vi "Main.vi"(8 "error in (no error)":errorcluster, 11 "DAQMH121119OrcaFlashBase in":refnum<class "DAQOrcaFlash.lvclass">) -> (0 "error out":errorcluster, 3 "component":refnum<class "DAQOrcaFlash.lvclass">)   [LabVIEW 2012, in "DAQOrcaFlash.lvclass"]
doc: "Main VI of the component."
uses:
  DAQOrcaFlash.lvclass
  binning.ctl
  DAQOrcaFlash.lvclass/DAQOrcaFlash.ctl
  <vilib>/Distrio/Murmex/InitialiseMessage/InitialiseMessage.lvclass
  <vilib>/Distrio/Murmex/Murmex/command_enum.ctl
  <vilib>/Distrio/Murmex/TerminateMessage/TerminateMessage.lvclass
  <vilib>/Distrio/Murmex/StartMessage/run mode enum.ctl
  <vilib>/Distrio/Murmex/StopMessage/StopMessage.lvclass
  <vilib>/Distrio/Murmex/StartMessage/StartMessage.lvclass
  <vilib>/Distrio/Murmex/ConfigureMessage/ConfigureMessage.lvclass
  <vilib>/Distrio/Murmex/Murmex/update_cluster.ctl
  class variable.vi
  <vilib>/Distrio/Murmex/Murmex/Set VI reference.vi
  <vilib>/Distrio/Murmex/Murmex/Set log reference.vi
  <vilib>/Distrio/Murmex/Murmex/Set configure at initialise.vi
  <vilib>/Distrio/Murmex/Murmex/Set relay start stop to observers.vi
  <vilib>/Distrio/Murmex/Murmex/Murmex.lvclass
  <vilib>/Distrio/Murmex/Message/Message.lvclass
panel:
  in  "button:configure":bool
  in  "button:quit":bool
  in  "terminate?":bool
  out "progress bar":sgl(slide) scale=0.0..1.0
  in  "Tab":T1(tab)
  in  "Rolling shutter pace":sgl[unit]=9.74436e-06 min=9.74436e-06 max=10 step=3.76e-09 format="%#_7g"
  out "Frames per second":dbl[unit]
  out "Virtual slit width":dbl[unit]
  in  "button:start_sweep":bool
  in  "y offset":u16 max=2048 step=4
  in  "x offset":u16 max=2048 step=4
  in  "y resolution":u16=2048 min=4 max=2048 step=4
  in  "x resolution":u16=2048 min=4 max=2048 step=4
  in  "binning":T2=1 items=["1x1"=1, "2x2"=2, "4x4"=4]
  in  "no. of frames":i32=1 min=1 step=1
  in  "line exposure time":dbl[unit]=0.1 caption="exposure time"
  in  "button:start focus":bool
  in  "File name":string
  in  "Subfolder levels":string[](array[string])
  in  "Custom saving path":bool
  in  "directory out":path
  in  "button:convert":bool
  out "filename":string
  in  "directory in":path
  in  "ID":string="orca"
  in  "log":string
  in  "button:AO":bool
  # "Convert here properietary file formats of Hamamatsu to TIFF format."
  # "Calculates the merit factor, \nused for Adaptive Optics (AO)"
  # "DAQMH121119OrcaFlash\n\nImplemented by:\nMarcel van 't Hoff\nUniversity of Florence, Ital\n\nThis component support only the Hamamatsu Orca Flash 4.0"
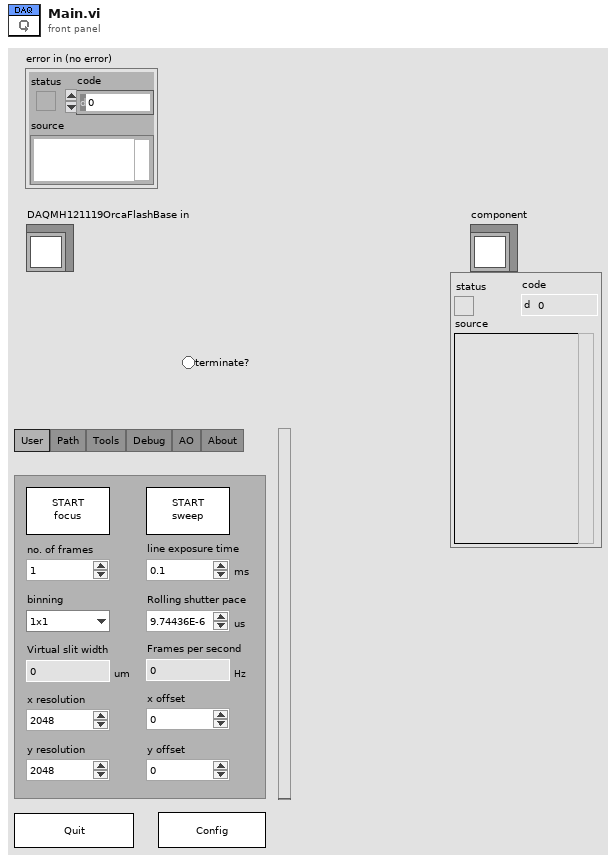
[diagram p1: front panel]
types:
  T1 = enum32{"User", "Path", "Tools", "Debug", "AO", "About"}
  T2 = typedef "DAQOrcaFlash.lvclass/binning.ctl" = u16
  T3 = typedef "Murmex.lvlib/Murmex.lvclass/command_enum.ctl" = enum16{"null", "initialise", "reset", "terminate", "acknowledge", "update", "inspect", "inform", "proceed", "start", "stop", "fetch", "configure", "generic"}
  T4 = typedef "Murmex.lvlib/StartMessage.lvclass/run mode enum.ctl" = enum16{"infinite", "finite"}
  T5 = typedef "Murmex.lvlib/Murmex.lvclass/update_cluster.ctl" = cluster{"target ID":string, "key chains":string[], "values":variant[]}
  T6 = enum8{"Enabled", "Disabled", "Disabled and Grayed Out"}
  T7 = typedef "Murmex.lvclass/command_enum.ctl" = enum16{"null", "initialise", "reset", "terminate", "acknowledge", "update", "inspect", "inform", "proceed", "start", "stop", "fetch", "configure", "generic"}
  T8 = typedef "Murmex.lvclass/Event type enumerations.ctl" = enum16{"before", "after"}
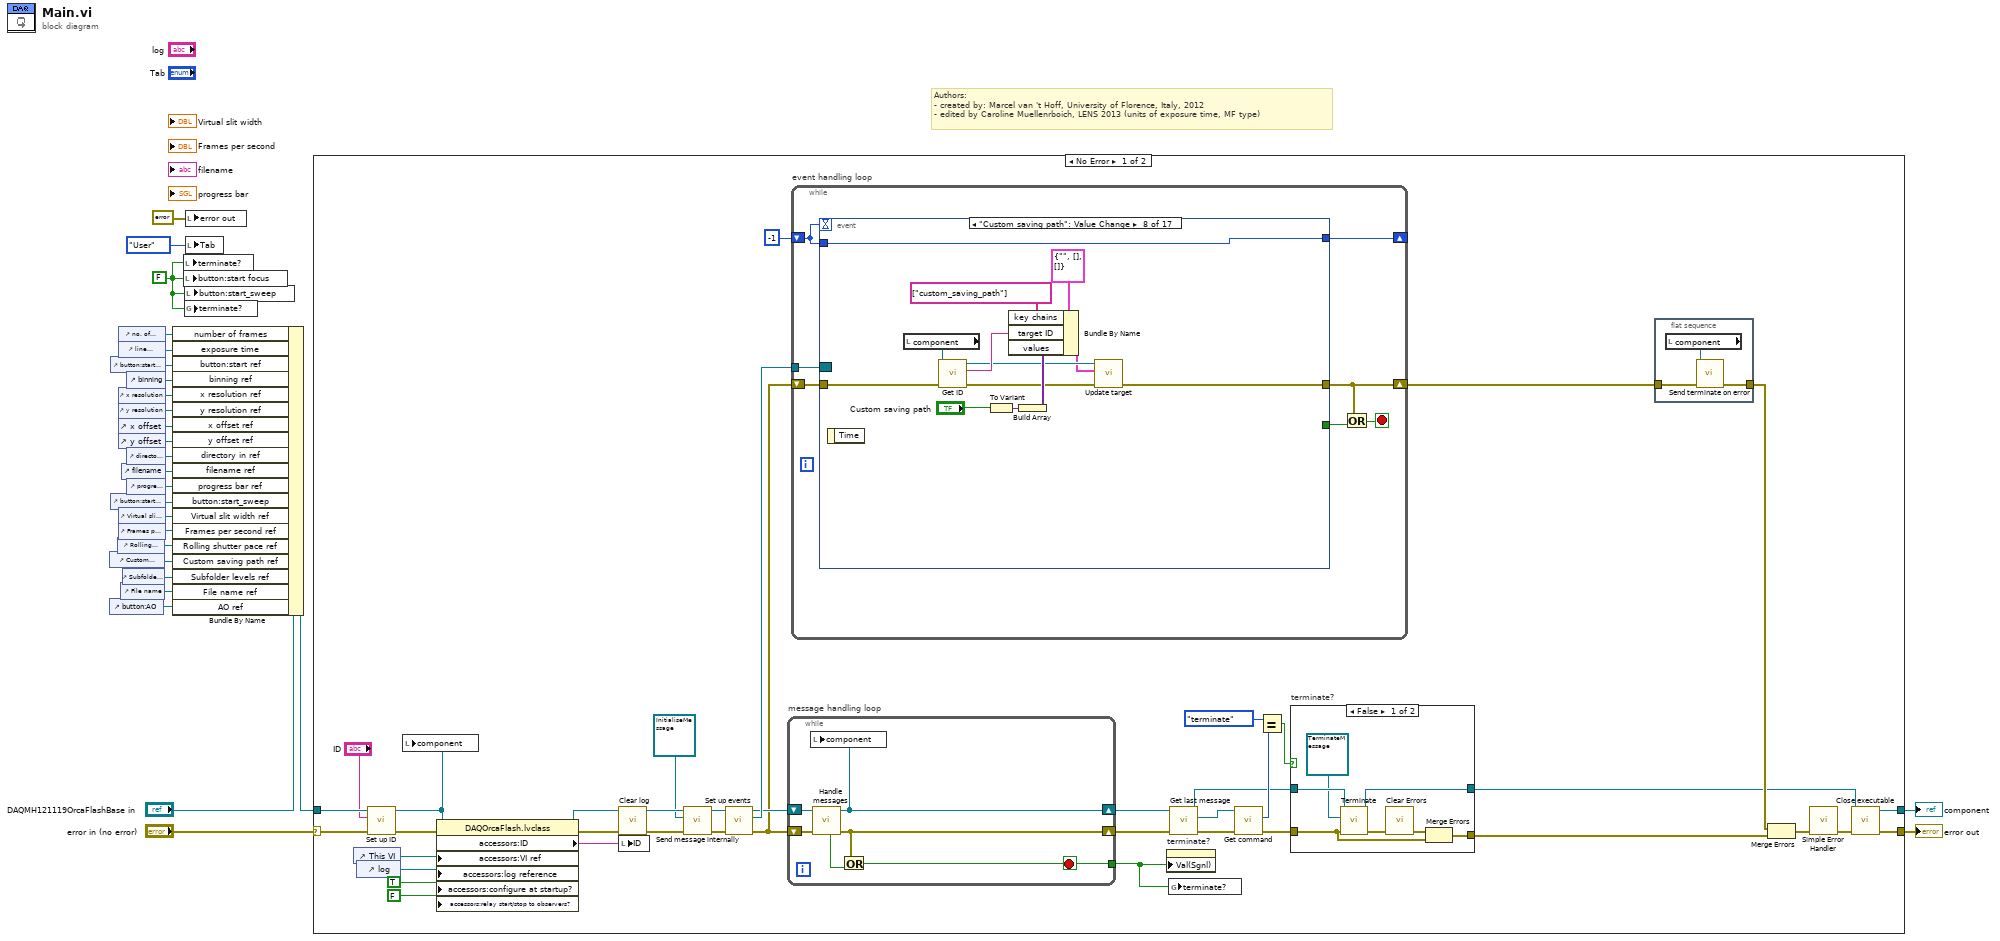
[diagram p0: block diagram]
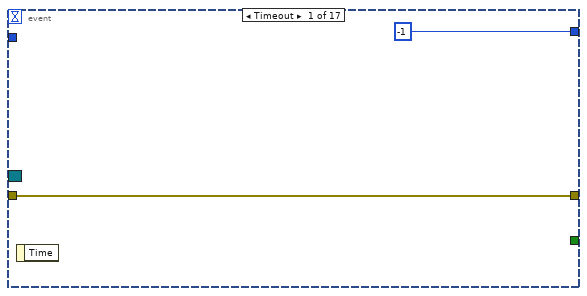
[diagram p3: hidden frame]
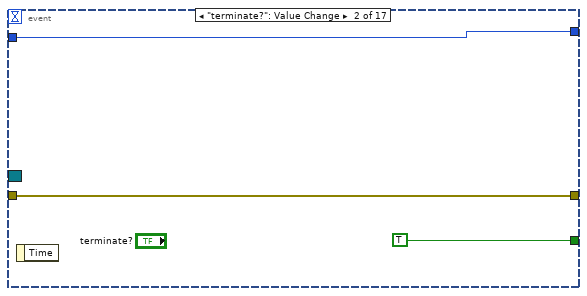
[diagram p4: hidden frame]
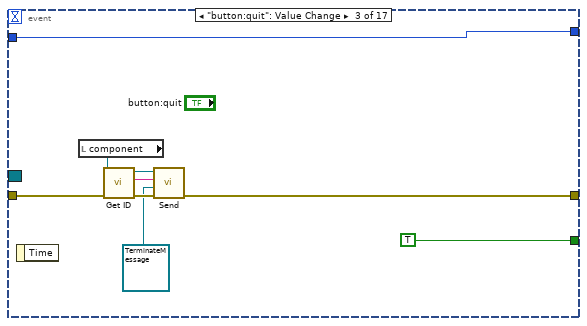
[diagram p5: hidden frame]
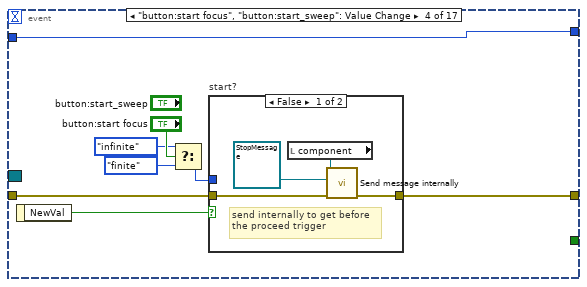
[diagram p6: hidden frame]
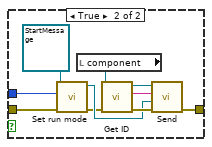
[diagram p7: hidden frame]
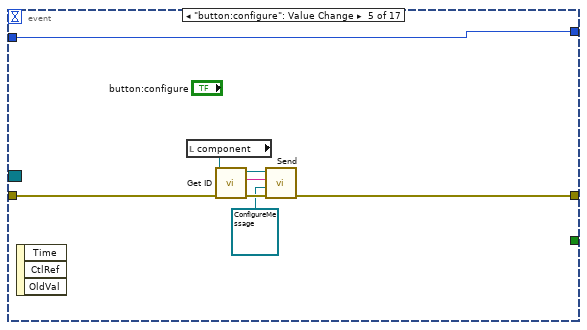
[diagram p8: hidden frame]
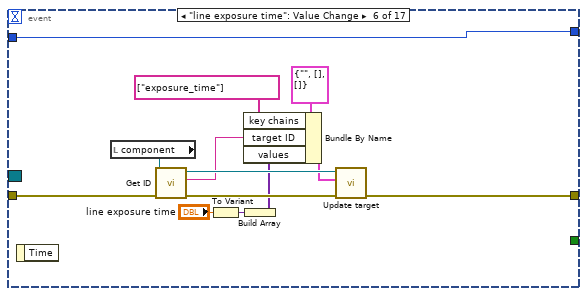
[diagram p9: hidden frame]
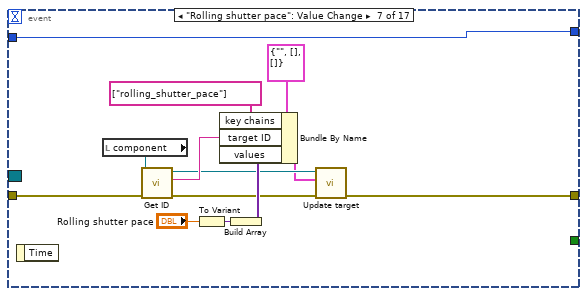
[diagram p10: hidden frame]
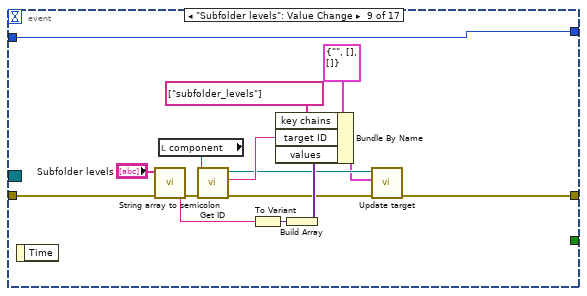
[diagram p11: hidden frame]
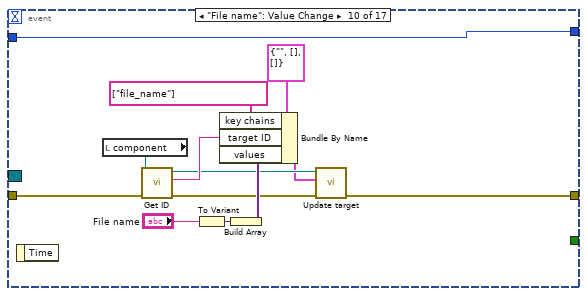
[diagram p12: hidden frame]
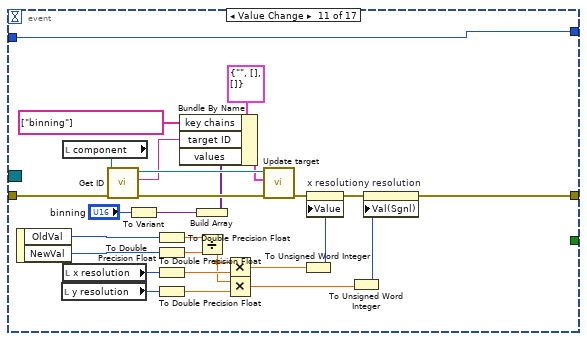
[diagram p13: hidden frame]
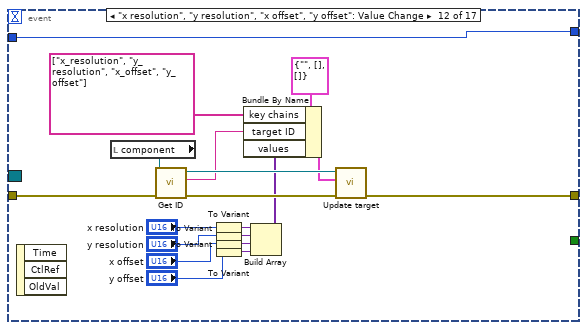
[diagram p14: hidden frame]
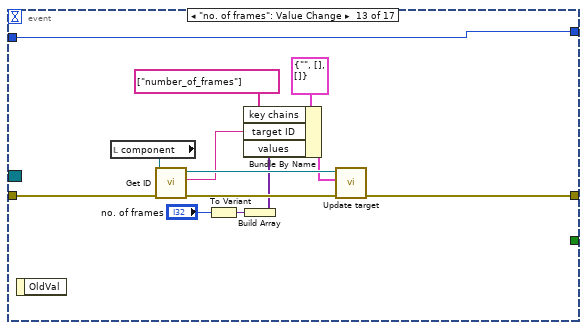
[diagram p15: hidden frame]
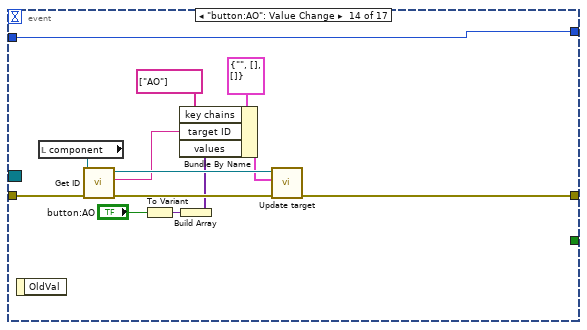
[diagram p16: hidden frame]
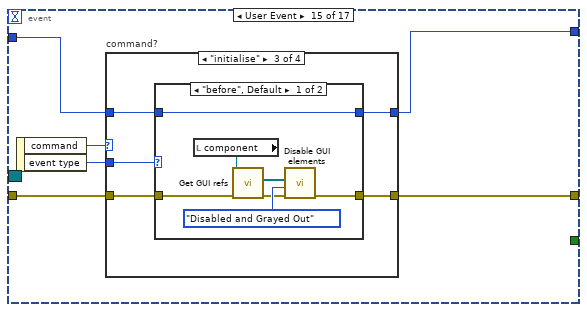
[diagram p17: hidden frame]
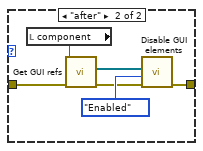
[diagram p19: hidden frame]
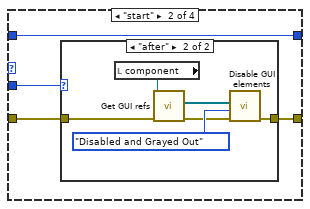
[diagram p20: hidden frame]
diagram:
  w9 = FALSE ("terminate?")
  # "Authors: \n- created by: Marcel van 't Hoff, University of Florence, Italy, 2012\n- edited by Caroline Muellenrboich, LENS 2013 (units of exposure time, MF type)"
  n1 = control-ref of="button:AO"() -> (w1:refnum<vi>)
  n2 = control-ref of="Custom saving path"() -> (w3:refnum<vi>)
  n3 = control-ref of="button:start focus"() -> (w20:refnum<vi>)
  n4 = control-ref of="button:start_sweep"() -> (w10:refnum<vi>)
  n5 = control-ref of="Rolling shutter pace"() -> (w6:refnum<vi>)
  n6 = control-ref of="no. of frames"() -> (w21:refnum<vi>)
  n7 = control-ref of="line exposure time"() -> (w22:refnum<vi>)
  n8 = control-ref of="x resolution"() -> (w18:refnum<vi>)
  n9 = control-ref of="y resolution"() -> (w17:refnum<vi>)
  n10 = control-ref of="x offset"() -> (w16:refnum<vi>)
  n11 = control-ref of="y offset"() -> (w15:refnum<vi>)
  n12 = control-ref of="Virtual slit width"() -> (w8:refnum<vi>)
  n13 = control-ref of="Frames per second"() -> (w7:refnum<vi>)
  n14 = control-ref of="File name"() -> (w5:refnum<vi>)
  n15 = control-ref of="filename"() -> (w13:refnum<vi>)
  n16 = control-ref of="Subfolder levels"() -> (w4:refnum<vi>)
  n17 = control-ref of="binning"() -> (w19:refnum<vi>)
  n18 = control-ref of="directory in"() -> (w14:refnum<vi>)
  n19 = control-ref of="progress bar"() -> (w12:refnum<vi>)
  n20 = Bundle By Name(cluster="DAQMH121119OrcaFlashBase in", "number of frames"=w21, "exposure time"=w22, "button:start ref"=w20, "binning ref"=w19, "x resolution ref"=w18, "y resolution ref"=w17, "x offset ref"=w16, "y offset ref"=w15, "directory in ref"=w14, "filename ref"=w13, "progress bar ref"=w12, "button:start_sweep"=w10, "Virtual slit width ref"=w8, "Frames per second ref"=w7, "Rolling shutter pace ref"=w6, "Custom saving path ref"=w3, "Subfolder levels ref"=w4, "File name ref"=w5, "AO ref"=w1) -> (w23:refnum<class "DAQOrcaFlash.lvclass">)
  n21 = local write "terminate?"(w9) -> ()
  n22 = local write "button:start focus"(w9) -> ()
  n23 = local write "button:start_sweep"(w9) -> ()
  n24 = global write "class variable.vi" "terminate?"(w9) -> ()
  n25 = local write "error out"(errorcluster {"status"=FALSE, "code"=0, "source"=""} ("error out")) -> ()
  n26 = local write "Tab"(T1."User" ("Tab")) -> ()
  n27 = case shown="No Error" "error in (no error)" {
    selector: "error in (no error)" -> [w60 w340]
    tunnel: [w55 w340] -> w26
    tunnel: [w54 w339] -> w25
    tunnel: w23 -> [w61 w339]
    frame No Error {
      n28 = control-ref of="This VI"() -> (w50:refnum<vi>)
      n29 = control-ref of="log"() -> (w49:refnum<vi>)
      n30 = call <vilib>:"Set up ID.vi"("error in (no error)"=w60, "component ID"="ID", "MurmexBase in"=w61) -> ("error out"=w52:errorcluster, "MurmexBase out"=w40:refnum<class "DAQOrcaFlash.lvclass">)  [unwired: 6 in, 1 out]
      n31 = local write "component"(w40) -> ()
      n32 = property class="DAQOrcaFlash.lvclass"(reference=w40, error in=w52, "accessors:VI ref"=w50, "accessors:log reference"=w49, "accessors:configure at startup?"=TRUE ("configure at startup?"), "accessors:relay start/stop to observers?"=FALSE ("relay start/stop to observers?")) -> (reference out=w47:refnum<class "DAQOrcaFlash.lvclass">, error out=w48:errorcluster, "accessors:ID"=w51:string)
      n33 = call <vilib>:"Clear log.vi"("error in (no error)"=w48, "MurmexBase in"=w47) -> ("error out"=w62:errorcluster, "MurmexBase out"=w66:refnum<class "DAQOrcaFlash.lvclass">)  [unwired: 8 in]
      n34 = local write "ID"(w51) -> ()
      n35 = call <vilib>:"Send message internally.vi"("error in (no error)"=w62, "Message"=refnum<class "InitialiseMessage.lvclass"> refnum ("Distrio Murmex 1.0:InitialiseMessage"), "Murmex in"=w66) -> ("error out"=w58:errorcluster, "Murmex out"=w57:refnum<class "DAQOrcaFlash.lvclass">)  [unwired: 7 in]
      n36 = call <vilib>:"Set up events.vi"("error in (no error)"=w58, "MurmexBase in"=w57) -> ("error out"=w29:errorcluster, "Event Registration Refnum"=w64:refnum<event-registration>, "MurmexBase out"=w31:refnum<class "DAQOrcaFlash.lvclass">)  [unwired: 7 in]
      n37 = while "message handling loop" {
        shift-right: [w334] -> w37
        shift-left: w29 -> [w336]
        shift-right: [w333] -> w39
        shift-left: w31 -> [w338]
        tunnel: [w335] -> w30
        stop <- w335 stop-if-true
        n38 = call <vilib>:"Handle messages.vi"("error in (no error)"=w336, "Murmex in"=w338) -> ("error out"=w334:errorcluster, "Murmex out"=w333:refnum<class "DAQOrcaFlash.lvclass">, "terminated?"=w337:bool)  [unwired: 7 in]
        n39 = local write "component"(w333) -> ()
        n40 = Or(x=w334, y=w337) -> (x .or. y?=w335:bool)
      }
      n41 = while "event handling loop" {
        shift-right: [w85] -> _
        shift-left: -1 -> [w84]
        tunnel: w64 -> [w82]
        shift-right: [w81] -> w63
        shift-left: w29 -> [w83]
        stop <- w79 stop-if-true
        n42 = event shown="[7] \"Custom saving path\": Value Change" {
          selector: w82 -> [_ _ _ _ _ _ _ _ _ _ _ _ _ _ _ _ _]
          dyn-events: _ -> [_ _ _ _ _ _ _ _ _ _ _ _ _ _ _ _ _]
          timeout: w84 -> [_ _ _ _ _ _ _ _ _ _ _ _ _ _ _ _ _]
          tunnel: [-1 w90 w99 w107 w129 w142 w155 w168 w183 w196 w224 w243 w256 w269 w271 w321 w332] -> w85
          tunnel: w84 -> [_ w90 w99 w107 w129 w142 w155 w168 w183 w196 w224 w243 w256 w269 w272 w321 w332]
          tunnel: w83 -> [w86 w89 w92 w106 w125 w141 w154 w167 w172 w195 w223 w242 w255 w268 w273 w320 w329]
          tunnel: [w86 w89 w94 w105 w124 w140 w147 w156 w176 w188 w206 w241 w254 w257 w274 w319 w322] -> w81
          tunnel: [_ TRUE TRUE _ _ _ _ _ _ _ _ _ _ _ _ _ _] -> w80
          event Timeout {
            n43 = event-data() -> ()  [unwired: 1 in, 1 out]
          }
          event "terminate?": Value Change {
            n44 = event-data() -> ()  [unwired: 1 in, 1 out]
          }
          event "button:quit": Value Change {
            n45 = event-data() -> ()  [unwired: 1 in, 1 out]
            n46 = local read "component"() -> (w97:refnum<class "DAQOrcaFlash.lvclass">)
            n47 = call <vilib>:"Get ID.vi"("error in (no error)"=w92, "Murmex in"=w97) -> ("error out"=w93:errorcluster, "component id"=w95:string, "Murmex out"=w96:refnum<class "DAQOrcaFlash.lvclass">)  [unwired: 7 in]
            n48 = call <vilib>:"Send.vi"("error in (no error)"=w93, "Message"=refnum<class "TerminateMessage.lvclass"> refnum ("Message in"), "recipient"=w95, "Murmex in"=w96) -> ("error out"=w94:errorcluster)  [unwired: 6 in, 1 out]
          }
          event "button:start focus", "button:start_sweep": Value Change {
            n49 = event-data() -> ("NewVal"=w102:bool)  [unwired: 1 in]
            n50 = Select(t=run_mode_enum."infinite" ("run mode"), s="button:start focus", f=run_mode_enum."finite" ("run mode")) -> (s? t:f=w103:T4)
            n51 = case "start?" shown="False" w102 {
              tunnel: [w110 w117] -> w105
              tunnel: w106 -> [w111 w114]
              tunnel: w103 -> [_ w112]
              frame False {
                # "send internally to get before\nthe proceed trigger"
                n52 = local read "component"() -> (w109:refnum<class "DAQOrcaFlash.lvclass">)
                n53 = call <vilib>:"Send message internally.vi"("error in (no error)"=w111, "Message"=refnum<class "StopMessage.lvclass"> refnum ("Distrio Murmex 1.0:StopMessage"), "Murmex in"=w109) -> ("error out"=w110:errorcluster)  [unwired: 7 in, 1 out]
              }
              frame True {
                n54 = call <vilib>:"Set run mode.vi"("error in (no error)"=w114, "run mode"=w112, "StartMessage in"=refnum<class "StartMessage.lvclass"> refnum ("Distrio Murmex 1.0:StartMessage")) -> ("error out"=w113:errorcluster, "StartMessage out"=w115:refnum<class "StartMessage.lvclass">)  [unwired: 7 in]
                n55 = local read "component"() -> (w121:refnum<class "DAQOrcaFlash.lvclass">)
                n56 = call <vilib>:"Get ID.vi"("error in (no error)"=w113, "Murmex in"=w121) -> ("error out"=w118:errorcluster, "component id"=w119:string, "Murmex out"=w120:refnum<class "DAQOrcaFlash.lvclass">)  [unwired: 7 in]
                n57 = call <vilib>:"Send.vi"("error in (no error)"=w118, "Message"=w115, "recipient"=w119, "Murmex in"=w120) -> ("error out"=w117:errorcluster)  [unwired: 6 in, 1 out]
              }
            }
          }
          event "button:configure": Value Change {
            n58 = event-data() -> ()  [unwired: 1 in, 3 out]
            n59 = local read "component"() -> (w123:refnum<class "DAQOrcaFlash.lvclass">)
            n60 = call <vilib>:"Get ID.vi"("error in (no error)"=w125, "Murmex in"=w123) -> ("error out"=w126:errorcluster, "component id"=w127:string, "Murmex out"=w128:refnum<class "DAQOrcaFlash.lvclass">)  [unwired: 7 in]
            n61 = call <vilib>:"Send.vi"("error in (no error)"=w126, "Message"=refnum<class "ConfigureMessage.lvclass"> refnum ("ConfigureMessage"), "recipient"=w127, "Murmex in"=w128) -> ("error out"=w124:errorcluster)  [unwired: 6 in, 1 out]
          }
          event "line exposure time": Value Change {
            n62 = event-data() -> ()  [unwired: 1 in, 1 out]
            n63 = local read "component"() -> (w139:refnum<class "DAQOrcaFlash.lvclass">)
            n64 = call <vilib>:"Get ID.vi"("error in (no error)"=w141, "Murmex in"=w139) -> ("error out"=w137:errorcluster, "component id"=w134:string, "Murmex out"=w138:refnum<class "DAQOrcaFlash.lvclass">)  [unwired: 7 in]
            n65 = To Variant(anything="line exposure time") -> (Variant=w132:variant)
            n66 = Build Array(w132) -> (w131:variant[])
            n67 = Bundle By Name(cluster=T5 {"target ID"="", "key chains"=[], "values"=[]} ("update cluster"), "key chains"=string[] ["exposure_time"], "target ID"=w134, "values"=w131) -> (w135:T5)
            n68 = call <vilib>:"Update target.vi"("error in (no error)"=w137, "update cluster"=w135, "MurmexBase in"=w138) -> ("error out"=w140:errorcluster)  [unwired: 7 in, 1 out]
          }
          event "Rolling shutter pace": Value Change {
            n69 = event-data() -> ()  [unwired: 1 in, 1 out]
            n70 = local read "component"() -> (w152:refnum<class "DAQOrcaFlash.lvclass">)
            n71 = call <vilib>:"Get ID.vi"("error in (no error)"=w154, "Murmex in"=w152) -> ("error out"=w148:errorcluster, "component id"=w151:string, "Murmex out"=w146:refnum<class "DAQOrcaFlash.lvclass">)  [unwired: 7 in]
            n72 = To Variant(anything="Rolling shutter pace") -> (Variant=w153:variant)
            n73 = Build Array(w153) -> (w149:variant[])
            n74 = Bundle By Name(cluster=T5 {"target ID"="", "key chains"=[], "values"=[]} ("update cluster"), "key chains"=string[] ["rolling_shutter_pace"], "target ID"=w151, "values"=w149) -> (w144:T5)
            n75 = call <vilib>:"Update target.vi"("error in (no error)"=w148, "update cluster"=w144, "MurmexBase in"=w146) -> ("error out"=w147:errorcluster)  [unwired: 7 in, 1 out]
          }
          event "Custom saving path": Value Change {
            n76 = event-data() -> ()  [unwired: 1 in, 1 out]
            n77 = local read "component"() -> (w165:refnum<class "DAQOrcaFlash.lvclass">)
            n78 = call <vilib>:"Get ID.vi"("error in (no error)"=w167, "Murmex in"=w165) -> ("error out"=w161:errorcluster, "component id"=w164:string, "Murmex out"=w160:refnum<class "DAQOrcaFlash.lvclass">)  [unwired: 7 in]
            n79 = To Variant(anything="Custom saving path") -> (Variant=w166:variant)
            n80 = Build Array(w166) -> (w162:variant[])
            n81 = Bundle By Name(cluster=T5 {"target ID"="", "key chains"=[], "values"=[]} ("update cluster"), "key chains"=string[] ["custom_saving_path"], "target ID"=w164, "values"=w162) -> (w158:T5)
            n82 = call <vilib>:"Update target.vi"("error in (no error)"=w161, "update cluster"=w158, "MurmexBase in"=w160) -> ("error out"=w156:errorcluster)  [unwired: 7 in, 1 out]
          }
          event "Subfolder levels": Value Change {
            n83 = event-data() -> ()  [unwired: 1 in, 1 out]
            n84 = call "String array to semicolon.vi"("error in"=w172, "String array"="Subfolder levels") -> ("error out"=w171:errorcluster, "Semicolon string"=w170:string)  [unwired: 8 in]
            n85 = local read "component"() -> (w181:refnum<class "DAQOrcaFlash.lvclass">)
            n86 = call <vilib>:"Get ID.vi"("error in (no error)"=w171, "Murmex in"=w181) -> ("error out"=w177:errorcluster, "component id"=w180:string, "Murmex out"=w175:refnum<class "DAQOrcaFlash.lvclass">)  [unwired: 7 in]
            n87 = To Variant(anything=w170) -> (Variant=w182:variant)
            n88 = Build Array(w182) -> (w178:variant[])
            n89 = Bundle By Name(cluster=T5 {"target ID"="", "key chains"=[], "values"=[]} ("update cluster"), "key chains"=string[] ["subfolder_levels"], "target ID"=w180, "values"=w178) -> (w173:T5)
            n90 = call <vilib>:"Update target.vi"("error in (no error)"=w177, "update cluster"=w173, "MurmexBase in"=w175) -> ("error out"=w176:errorcluster)  [unwired: 7 in, 1 out]
          }
          event "File name": Value Change {
            n91 = event-data() -> ()  [unwired: 1 in, 1 out]
            n92 = local read "component"() -> (w193:refnum<class "DAQOrcaFlash.lvclass">)
            n93 = call <vilib>:"Get ID.vi"("error in (no error)"=w195, "Murmex in"=w193) -> ("error out"=w189:errorcluster, "component id"=w192:string, "Murmex out"=w187:refnum<class "DAQOrcaFlash.lvclass">)  [unwired: 7 in]
            n94 = To Variant(anything="File name") -> (Variant=w194:variant)
            n95 = Build Array(w194) -> (w190:variant[])
            n96 = Bundle By Name(cluster=T5 {"target ID"="", "key chains"=[], "values"=[]} ("update cluster"), "key chains"=string[] ["file_name"], "target ID"=w192, "values"=w190) -> (w185:T5)
            n97 = call <vilib>:"Update target.vi"("error in (no error)"=w189, "update cluster"=w185, "MurmexBase in"=w187) -> ("error out"=w188:errorcluster)  [unwired: 7 in, 1 out]
          }
          event Value Change {
            n98 = event-data() -> ("OldVal"=w201:T2, "NewVal"=w200:T2)  [unwired: 1 in]
            n99 = local read "y resolution"() -> (w214:u16)
            n100 = local read "component"() -> (w222:refnum<class "DAQOrcaFlash.lvclass">)
            n101 = local read "x resolution"() -> (w213:u16)
            n102 = call <vilib>:"Get ID.vi"("error in (no error)"=w223, "Murmex in"=w222) -> ("error out"=w220:errorcluster, "component id"=w217:string, "Murmex out"=w221:refnum<class "DAQOrcaFlash.lvclass">)  [unwired: 7 in]
            n103 = To Variant(anything="binning") -> (Variant=w209:variant)
            n104 = To Double Precision Float(number=w201) -> (double precision float=w199:dbl)
            n105 = To Double Precision Float(number=w200) -> (double precision float=w198:dbl)
            n106 = To Double Precision Float(number=w213) -> (double precision float=w210:dbl)
            n107 = To Double Precision Float(number=w214) -> (double precision float=w211:dbl)
            n108 = Build Array(w209) -> (w215:variant[])
            n109 = Bundle By Name(cluster=T5 {"target ID"="", "key chains"=[], "values"=[]} ("update cluster"), "key chains"=string[] ["binning"], "target ID"=w217, "values"=w215) -> (w218:T5)
            n110 = Divide(x=w199, y=w198) -> (x/y=w197:dbl)
            n111 = Multiply(x=w197, y=w210) -> (x*y=w207:dbl)
            n112 = Multiply(x=w197, y=w211) -> (x*y=w208:dbl)
            n113 = call <vilib>:"Update target.vi"("error in (no error)"=w220, "update cluster"=w218, "MurmexBase in"=w221) -> ("error out"=w205:errorcluster)  [unwired: 7 in, 1 out]
            n114 = To Unsigned Word Integer(number=w207) -> (unsigned 16bit integer=w204:u16)
            n115 = property on="x resolution" class="DigNum (strict)"(error in=w205, "Value"=w204) -> (error out=w202:errorcluster)  [unwired: 1 in, 1 out]
            n116 = To Unsigned Word Integer(number=w208) -> (unsigned 16bit integer=w203:u16)
            n117 = property on="y resolution" class="DigNum (strict)"(error in=w202, "Val(Sgnl)"=w203) -> (error out=w206:errorcluster)  [unwired: 1 in, 1 out]
          }
          event "x resolution", "y resolution", "x offset", "y offset": Value Change {
            n118 = event-data() -> ()  [unwired: 1 in, 3 out]
            n119 = local read "component"() -> (w240:refnum<class "DAQOrcaFlash.lvclass">)
            n120 = call <vilib>:"Get ID.vi"("error in (no error)"=w242, "Murmex in"=w240) -> ("error out"=w238:errorcluster, "component id"=w235:string, "Murmex out"=w239:refnum<class "DAQOrcaFlash.lvclass">)  [unwired: 7 in]
            n121 = To Variant(anything="x resolution") -> (Variant=w228:variant)
            n122 = To Variant(anything="y resolution") -> (Variant=w227:variant)
            n123 = To Variant(anything="x offset") -> (Variant=w226:variant)
            n124 = To Variant(anything="y offset") -> (Variant=w225:variant)
            n125 = Build Array(w228, w227, w226, w225) -> (w229:variant[])
            n126 = Bundle By Name(cluster=T5 {"target ID"="", "key chains"=[], "values"=[]} ("update cluster"), "key chains"=string[] ["x_resolution", "y_resolution", "x_offset", "y_offset"], "target ID"=w235, "values"=w229) -> (w236:T5)
            n127 = call <vilib>:"Update target.vi"("error in (no error)"=w238, "update cluster"=w236, "MurmexBase in"=w239) -> ("error out"=w241:errorcluster)  [unwired: 7 in, 1 out]
          }
          event "no. of frames": Value Change {
            n128 = event-data() -> ()  [unwired: 1 in, 1 out]
            n129 = local read "component"() -> (w253:refnum<class "DAQOrcaFlash.lvclass">)
            n130 = call <vilib>:"Get ID.vi"("error in (no error)"=w255, "Murmex in"=w253) -> ("error out"=w251:errorcluster, "component id"=w248:string, "Murmex out"=w252:refnum<class "DAQOrcaFlash.lvclass">)  [unwired: 7 in]
            n131 = To Variant(anything="no. of frames") -> (Variant=w244:variant)
            n132 = Build Array(w244) -> (w246:variant[])
            n133 = Bundle By Name(cluster=T5 {"target ID"="", "key chains"=[], "values"=[]} ("update cluster"), "key chains"=string[] ["number_of_frames"], "target ID"=w248, "values"=w246) -> (w249:T5)
            n134 = call <vilib>:"Update target.vi"("error in (no error)"=w251, "update cluster"=w249, "MurmexBase in"=w252) -> ("error out"=w254:errorcluster)  [unwired: 7 in, 1 out]
          }
          event "button:AO": Value Change {
            n135 = event-data() -> ()  [unwired: 1 in, 1 out]
            n136 = local read "component"() -> (w267:refnum<class "DAQOrcaFlash.lvclass">)
            n137 = call <vilib>:"Get ID.vi"("error in (no error)"=w268, "Murmex in"=w267) -> ("error out"=w265:errorcluster, "component id"=w258:string, "Murmex out"=w266:refnum<class "DAQOrcaFlash.lvclass">)  [unwired: 7 in]
            n138 = To Variant(anything="button:AO") -> (Variant=w260:variant)
            n139 = Build Array(w260) -> (w261:variant[])
            n140 = Bundle By Name(cluster=T5 {"target ID"="", "key chains"=[], "values"=[]} ("update cluster"), "key chains"=string[] ["AO"], "target ID"=w258, "values"=w261) -> (w263:T5)
            n141 = call <vilib>:"Update target.vi"("error in (no error)"=w265, "update cluster"=w263, "MurmexBase in"=w266) -> ("error out"=w257:errorcluster)  [unwired: 7 in, 1 out]
          }
          event User Event {
            n142 = event-data() -> ("command"=w275:T7, "event type"=w270:T8)  [unwired: 1 in]
            n143 = case "command?" shown="\"initialise\"" w275 {
              tunnel: [w279 w290 w301 w315] -> w274
              tunnel: w273 -> [w278 w289 w302 w315]
              tunnel: [w277 w288 w300 w314] -> w271
              tunnel: w272 -> [w277 w288 w299 w314]
              tunnel: w270 -> [w276 w287 w298 _]
              frame "stop" {
                n144 = case shown="\"before\", Default" w276 {
                  tunnel: [w280 w286] -> w279
                  tunnel: w278 -> [w280 w283]
                  frame "before", Default {
                  }
                  frame "after" {
                    n145 = local read "component"() -> (w284:refnum<class "DAQOrcaFlash.lvclass">)
                    n146 = call "Get GUI refs.vi"("error in (no error)"=w283, "DAQMH121119OrcaFlash in"=w284) -> ("error out"=w282:errorcluster, "Array"=w281:refnum<vi>[])  [unwired: 7 in, 1 out]
                    n147 = call <vilib>:"Disable GUI elements.vi"("error in (no error)"=w282, "enabled state"=T6."Enabled", "control refs"=w281) -> ("error out"=w286:errorcluster)  [unwired: 8 in]
                  }
                }
              }
              frame "start" {
                n148 = case shown="\"after\"" w287 {
                  tunnel: [w291 w297] -> w290
                  tunnel: w289 -> [w291 w295]
                  frame "before", Default {
                  }
                  frame "after" {
                    n149 = local read "component"() -> (w292:refnum<class "DAQOrcaFlash.lvclass">)
                    n150 = call "Get GUI refs.vi"("error in (no error)"=w295, "DAQMH121119OrcaFlash in"=w292) -> ("error out"=w294:errorcluster, "Array"=w293:refnum<vi>[])  [unwired: 7 in, 1 out]
                    n151 = call <vilib>:"Disable GUI elements.vi"("error in (no error)"=w294, "enabled state"=T6."Disabled and Grayed Out", "control refs"=w293) -> ("error out"=w297:errorcluster)  [unwired: 8 in]
                  }
                }
              }
              frame "initialise" {
                n152 = case shown="\"before\", Default" w298 {
                  tunnel: w302 -> [w304 w312]
                  tunnel: [w303 w311] -> w301
                  tunnel: [w309 -1] -> w300
                  tunnel: w299 -> [w309 _]
                  frame "before", Default {
                    n153 = local read "component"() -> (w305:refnum<class "DAQOrcaFlash.lvclass">)
                    n154 = call "Get GUI refs.vi"("error in (no error)"=w304, "DAQMH121119OrcaFlash in"=w305) -> ("error out"=w307:errorcluster, "Array"=w306:refnum<vi>[])  [unwired: 7 in, 1 out]
                    n155 = call <vilib>:"Disable GUI elements.vi"("error in (no error)"=w307, "enabled state"=T6."Disabled and Grayed Out", "control refs"=w306) -> ("error out"=w303:errorcluster)  [unwired: 8 in]
                  }
                  frame "after" {
                    n156 = local read "component"() -> (w313:refnum<class "DAQOrcaFlash.lvclass">)
                    n157 = call "Initialise parameters.vi"("error in (no error)"=w312, "DAQMH121119OrcaFlash in"=w313) -> ("error out"=w311:errorcluster)  [unwired: 8 in, 1 out]
                  }
                }
              }
              frame Default {
              }
            }
          }
          event "button:convert": Value Change {
            n158 = event-data() -> ()  [unwired: 1 in, 1 out]
            n159 = local read "component"() -> (w318:refnum<class "DAQOrcaFlash.lvclass">)
            n160 = call "Convert directory.vi"("error in (no error)"=w320, "directory out"="directory out", "directory in"="directory in", "DAQMH121119OrcaFlash in"=w318) -> ("error out"=w319:errorcluster)  [unwired: 6 in, 1 out]
          }
          event "directory in", "directory out": Value Change {
            n161 = event-data() -> ()  [unwired: 1 in, 1 out]
            n162 = local read "directory out"() -> (w331:path)
            n163 = local read "directory in"() -> (w328:path)
            n164 = call <vilib>:"Check if File or Folder Exists.vi"("error in (no error)"=w329, "path"=w331) -> ("error out"=w330:errorcluster, "file or folder exists?"=w326:bool)  [unwired: 7 in, 1 out]
            n165 = call <vilib>:"Check if File or Folder Exists.vi"("error in (no error)"=w330, "path"=w328) -> ("error out"=w323:errorcluster, "file or folder exists?"=w327:bool)  [unwired: 7 in, 1 out]
            n166 = And(x=w327, y=w326) -> (x .and. y?=w325:bool)
            n167 = call "bool_to_enable_state.vi"("boolean in"=w325) -> ("enabled status out"=w324:T6)  [unwired: 4 in]
            n168 = property on="button:convert" class="Bool"(error in=w323, "DisabledEnum"=w324) -> (error out=w322:errorcluster)  [unwired: 1 in, 1 out]
          }
        }
        n169 = Or(x=w81, y=w80) -> (x .or. y?=w79:bool)
      }
      n170 = property on="terminate?" class="Bool (strict)"("Val(Sgnl)"=w30) -> ()  [unwired: 2 in, 2 out]
      n171 = global write "class variable.vi" "terminate?"(w30) -> ()
      n172 = call <vilib>:"Get last message.vi"("error in (no error)"=w37, "MurmexBase in"=w39) -> ("error out"=w36:errorcluster, "Message"=w35:refnum<class "Message.lvclass">, "MurmexBase out"=w38:refnum<class "DAQOrcaFlash.lvclass">)  [unwired: 7 in]
      n173 = call <vilib>:"Get command.vi"("error in (no error)"=w36, "Message in"=w35) -> ("error out"=w43:errorcluster, "command"=w45:T3)  [unwired: 7 in, 1 out]
      n174 = Equal?(x=command_enum."terminate", y=w45) -> (x = y?=w41:bool)
      n175 = case "terminate?" shown="False" w41 {
        tunnel: w38 -> [w72 w75]
        tunnel: [w71 w75] -> w53
        tunnel: w43 -> [w70 w74]
        tunnel: [w68 w74] -> w42
        frame False {
          n176 = call-dynamic "Terminate.vi"("error in (no error)"=w70, "Message in"=refnum<class "TerminateMessage.lvclass"> refnum, "DAQMH121119OrcaFlash in"=w72) -> ("error out"=w73:errorcluster, "DAQMH121119OrcaFlash out"=w71:refnum<class "DAQOrcaFlash.lvclass">)  [unwired: 7 in]
          n177 = call <vilib>:"Clear Errors.vi"("error in (no error)"=w73) -> ("error out"=w69:errorcluster)  [unwired: 6 in]
          n178 = Merge Errors(w69, w70) -> (w68:errorcluster)
        }
        frame True {
        }
      }
      n179 = flat-sequence {
        tunnel: w63 -> [w78]
        tunnel: [w77] -> w56
        frame #0 {
          n180 = local read "component"() -> (w76:refnum<class "DAQOrcaFlash.lvclass">)
          n181 = call <vilib>:"Send terminate on error.vi"("error in (no error)"=w78, "Murmex in"=w76) -> ("error out"=w77:errorcluster)  [unwired: 8 in, 1 out]
        }
      }
      n182 = Merge Errors(w56, w42) -> (w33:errorcluster)
      n183 = call <vilib>:"Simple Error Handler.vi"("error in (no error)"=w33) -> ("error out"=w32:errorcluster)  [unwired: 4 in, 4 out]
      n184 = call <vilib>:"Close executable.vi"("error in (no error)"=w32, "MurmexBase in"=w53) -> ("error out"=w55:errorcluster, "MurmexBase out"=w54:refnum<class "DAQOrcaFlash.lvclass">)  [unwired: 8 in]
    }
    frame Error {
    }
  }
  "error out" <- w26
  "component" <- w25
